vi "Teste_OpenFile.vi"() -> ()   [LabVIEW 2013]
panel:
  in  "Inteiro 2":i32=25
  in  "Real 2":dbl format="%#_13g"
  in  "Inteiro":i32=25
  in  "Real":dbl format="%#_13g"
  in  "Arquivo":path
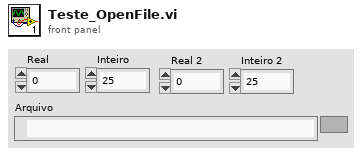
[diagram p1: front panel]
types:
  T1 = enum16{"open", "replace", "create", "open or create", "replace or create", "replace or create with confirmation"}
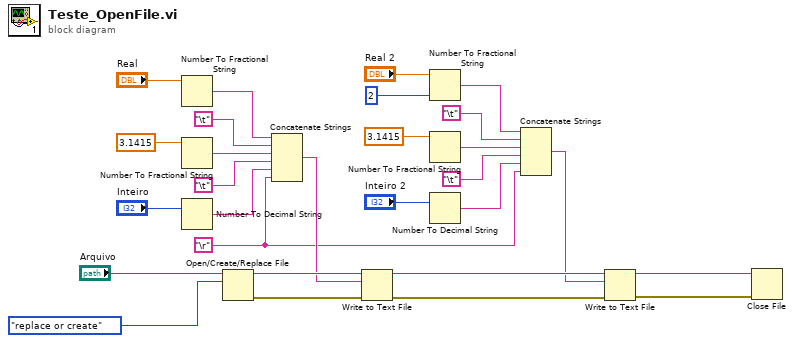
[diagram p0: block diagram]
diagram:
  w2 = "\r"
  n1 = Number To Fractional String(number="Real") -> (F-format string=w22:string)  [unwired: 3 in]
  n2 = Number To Fractional String(number=3.1415) -> (F-format string=w20:string)  [unwired: 3 in]
  n3 = Number To Decimal String(number="Inteiro") -> (decimal integer string=w17:string)  [unwired: 1 in]
  n4 = Open/Create/Replace File(file path (use dialog)="Arquivo", operation (0:open)=T1."replace or create") -> (refnum out=w26:refnum<file>, error out=w25:errorcluster)  [unwired: 4 in, 1 out]
  n5 = Concatenate Strings(w22, "\t", w20, "\t", w17, w2) -> (w16:string)
  n6 = Write to Text File(file (use dialog)=w26, text=w16, error in=w25) -> (refnum out=w15:refnum<file>, error out=w14:errorcluster)  [unwired: 1 in, 1 out]
  n7 = Number To Fractional String(number="Real 2", precision (6)=2) -> (F-format string=w9:string)  [unwired: 2 in]
  n8 = Number To Fractional String(number=3.1415) -> (F-format string=w7:string)  [unwired: 3 in]
  n9 = Number To Decimal String(number="Inteiro 2") -> (decimal integer string=w4:string)  [unwired: 1 in]
  n10 = Concatenate Strings(w9, "\t", w7, "\t", w4, w2) -> (w3:string)
  n11 = Write to Text File(file (use dialog)=w15, text=w3, error in=w14) -> (refnum out=w13:refnum<file>, error out=w12:errorcluster)  [unwired: 1 in, 1 out]
  n12 = Close File(refnum=w13, error in=w12) -> ()  [unwired: 2 out]
